vi "Alive_Check.vi"(10 "Timeout_msec":u32, 11 "Alv_cnt":u8) -> (2 "Timeout":bool, 3 "Error":bool)   [LabVIEW 2015]
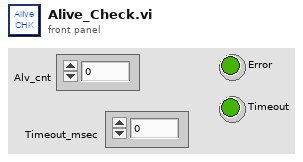
[diagram p1: front panel]
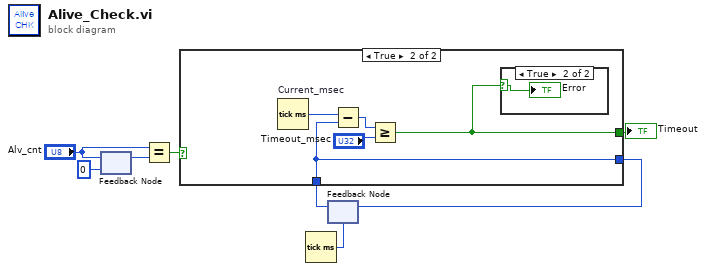
[diagram p0: block diagram]
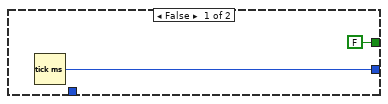
[diagram p2: hidden frame]
diagram:
  n1 = feedback #1(u8 0 ("Alv_cnt")) -> (w4:u8)
  n2 = feedback-in #1("Alv_cnt") -> ()
  n3 = Equal?(x="Alv_cnt", y=w4) -> (x = y?=w1:bool)
  n4 = Tick Count (ms) ("Current_msec")() -> (millisecond timer value=w7:u32)
  n5 = feedback #2(w7) -> (w2:u32)
  n6 = case shown="True" w1 {
    tunnel: [FALSE w11] -> w8
    tunnel: w2 -> [_ w12]
    tunnel: [w10 w12] -> w3
    frame False {
      n7 = Tick Count (ms)() -> (millisecond timer value=w10:u32)
    }
    frame True {
      n8 = Tick Count (ms) "Current_msec"() -> (millisecond timer value=w13:u32)
      n9 = Subtract(x=w13, y=w12) -> (x-y=w14:u32)
      n10 = Greater Or Equal?(x=w14, y="Timeout_msec") -> (x >= y?=w11:bool)
      n11 = case shown="True" w11 {
        selector: w11 -> [_ w16]
        frame False {
        }
        frame True {
          "Error" <- w16
        }
      }
    }
  }
  "Timeout" <- w8
  n12 = feedback-in #2(w3) -> ()
